vi "Update Rate.vi"(8 "Error In":errorcluster) -> (0 "Error Out":errorcluster, 1 "Interval [s]":dbl, 2 "Update Rate [1/s]":dbl)   [LabVIEW 2016]
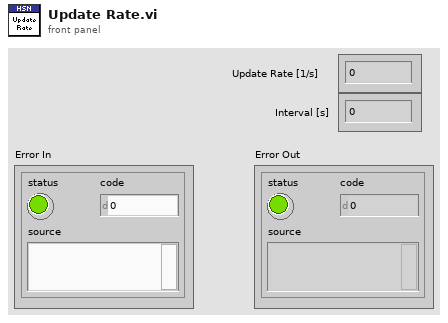
[diagram p1: front panel]
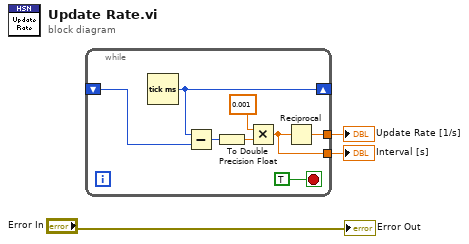
[diagram p0: block diagram]
diagram:
  n1 = while {
    tunnel: [w9] -> w3
    shift-right: [w5] -> _
    shift-left: _ -> [w7]
    tunnel: [w4] -> w2
    stop <- TRUE stop-if-true
    n2 = Tick Count (ms)() -> (millisecond timer value=w5:u32)
    n3 = Subtract(x=w5, y=w7) -> (x-y=w11:u32)
    n4 = To Double Precision Float(number=w11) -> (double precision float=w6:dbl)
    n5 = Multiply(x=0.001 ("y"), y=w6) -> (x*y=w4:dbl)
    n6 = Reciprocal(x=w4) -> (1/x=w9:dbl)
  }
  "Update Rate [1/s]" <- w3
  "Interval [s]" <- w2
  "Error Out" <- "Error In"
